vi "Reset After Waveform Acquisition.vi"(8 "error in (no error)":errorcluster, 10 "Channel Name":string, 11 "Scope in":refnum<class "Scope.lvclass">) -> (0 "error out":errorcluster, 3 "Scope out":refnum<class "Scope.lvclass">)   [LabVIEW 2015, in "Scope.lvclass"]
uses:
  Scope.lvclass
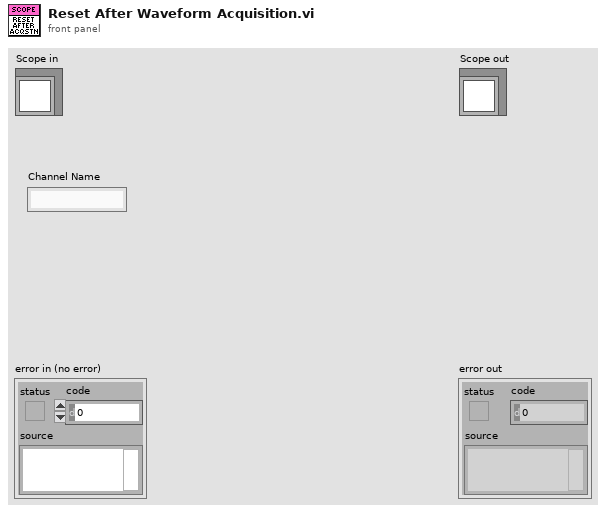
[diagram p1: front panel]
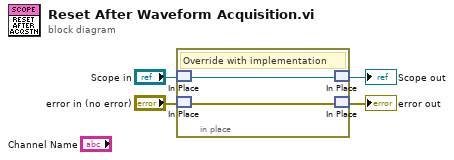
[diagram p0: block diagram]
diagram:
  n1 = in-place {
    # "Override with implementation"
    n2 = in-place-match #1("Scope in") -> (w6:refnum<class "Scope.lvclass">)
    n3 = in-place-match #2("error in (no error)") -> (w5:errorcluster)
    n4 = in-place-match #1(w6) -> (→"Scope out":refnum<class "Scope.lvclass">)
    n5 = in-place-match #2(w5) -> (→"error out":errorcluster)
  }
